vi "Node 2 - Error Handler.vi"(8 "Error In":errorcluster, 11 "State In":T1) -> (0 "Error Out":errorcluster, 3 "State Out":T1)   [LabVIEW 2018]
uses:
  Node 2 - States.ctl
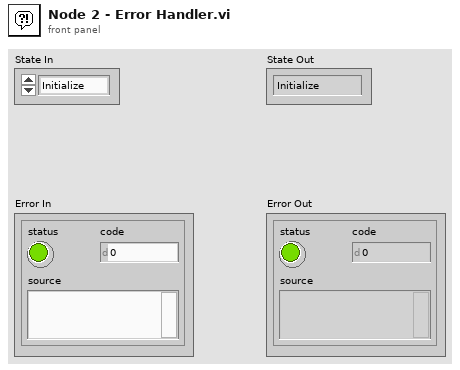
[diagram p1: front panel]
types:
  T1 = typedef "Node 2 - States.ctl" = enum16{"Initialize", "Read Pump State", "Toggle Pump", "Send HB", "Error", "Manual Mode"}
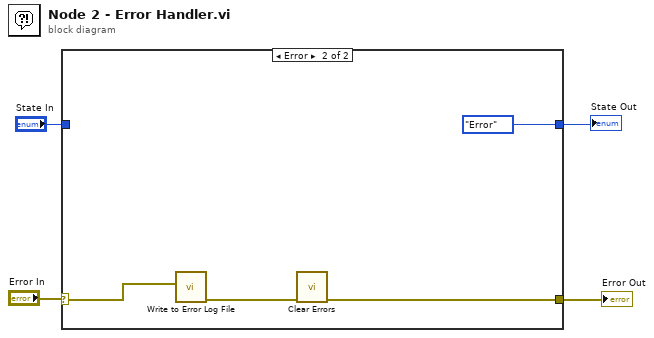
[diagram p0: block diagram]
diagram:
  n1 = case shown="Error" "Error In" {
    selector: "Error In" -> [w6 w10]
    tunnel: [w6 w8] -> w3
    tunnel: "State In" -> [w5 _]
    tunnel: [w5 Node_2_-_States."Error" ("State In")] -> w1
    frame No Error {
    }
    frame Error {
      n2 = call "Write to Error Log File.vi"("error in (no error)"=w10) -> ("Error Out"=w7:errorcluster)  [unwired: 10 in]
      n3 = call <vilib>:"Clear Errors.vi"("error in (no error)"=w7) -> ("error out"=w8:errorcluster)  [unwired: 5 in, 1 out]
    }
  }
  "State Out" <- w1
  "Error Out" <- w3
